vi "TestFileCreationAndWriting.vi"() -> ()   [LabVIEW 2014]
panel:
  in  "VME Configuration":T1={"Module Description"=["Bridge", "TDC", "Scaler", "Hodoscope QDC ", "Other QDC", "Digitizer 1", "Digitizer 2", ""], "Module Model"=["V2718", "V775", "V830", "V965A", "V965A", "V1729A", "1729A", ""], "Module Address"=[0, 4026597376, 4026662912, 4026728448, 4026793984, 4026859520, 4026925056]} {"Module Address" format="%.0x"}
  out "error out":errorcluster
  out "Average Write Time (ms)":dbl=11.54
  out "Max Write Time":u32=42
  in  "Number of Events":i32=100
  in  "QDC Info":T2={"Chanel Description"=["H0", "H1", "H2", "H3", "H4", "H5"], "Only Hodo?"=[TRUE, TRUE, TRUE, TRUE, TRUE, TRUE]}
  in  "Scaler Info":T2={"Chanel Description"=["H0", "H1", "H2", "H3", "H4", "H5", "TrigA", "TrigB", "TrigC", "TrigD", "Ch0", "Ch1", "Ch2", "Ch3", "Ch4", "Ch5", "Ch6", "Ch7"], "Only Hodo?"=[TRUE, TRUE, TRUE, TRUE, TRUE, TRUE, TRUE, TRUE, FALSE, FALSE, FALSE, FALSE, FALSE, FALSE, FALSE, FALSE, FALSE, FALSE]}
  in  "Digitizer Info":T2={"Chanel Description"=["Ch0", "Ch1", "Ch2", "Ch3", "Ch4", "Ch5", "Ch6", "Ch7"], "Only Hodo?"=[FALSE, FALSE, FALSE, FALSE, FALSE, FALSE, FALSE, FALSE]}
  in  "TDC Info":T2={"Chanel Description"=["H0", "H1", "H2", "H3", "H4", "H5", "TrigA", "TrigB", "TrigC", "TrigD"], "Only Hodo?"=[TRUE, TRUE, TRUE, TRUE, TRUE, TRUE, TRUE, TRUE, FALSE, FALSE]}
  in  "Trigger Bit Descriptions":string[](array[string])=["TrigA", "TrigB", "TrigC", "TrigD"]
  in  "Thermocouple Location":string[](array[string])=["In Dark Box", "In Room"]
  in  "HDF5 File Path":path=path "C:/Users/lbignell/Desktop/Control Software/HDF5/Dummy3.h5"
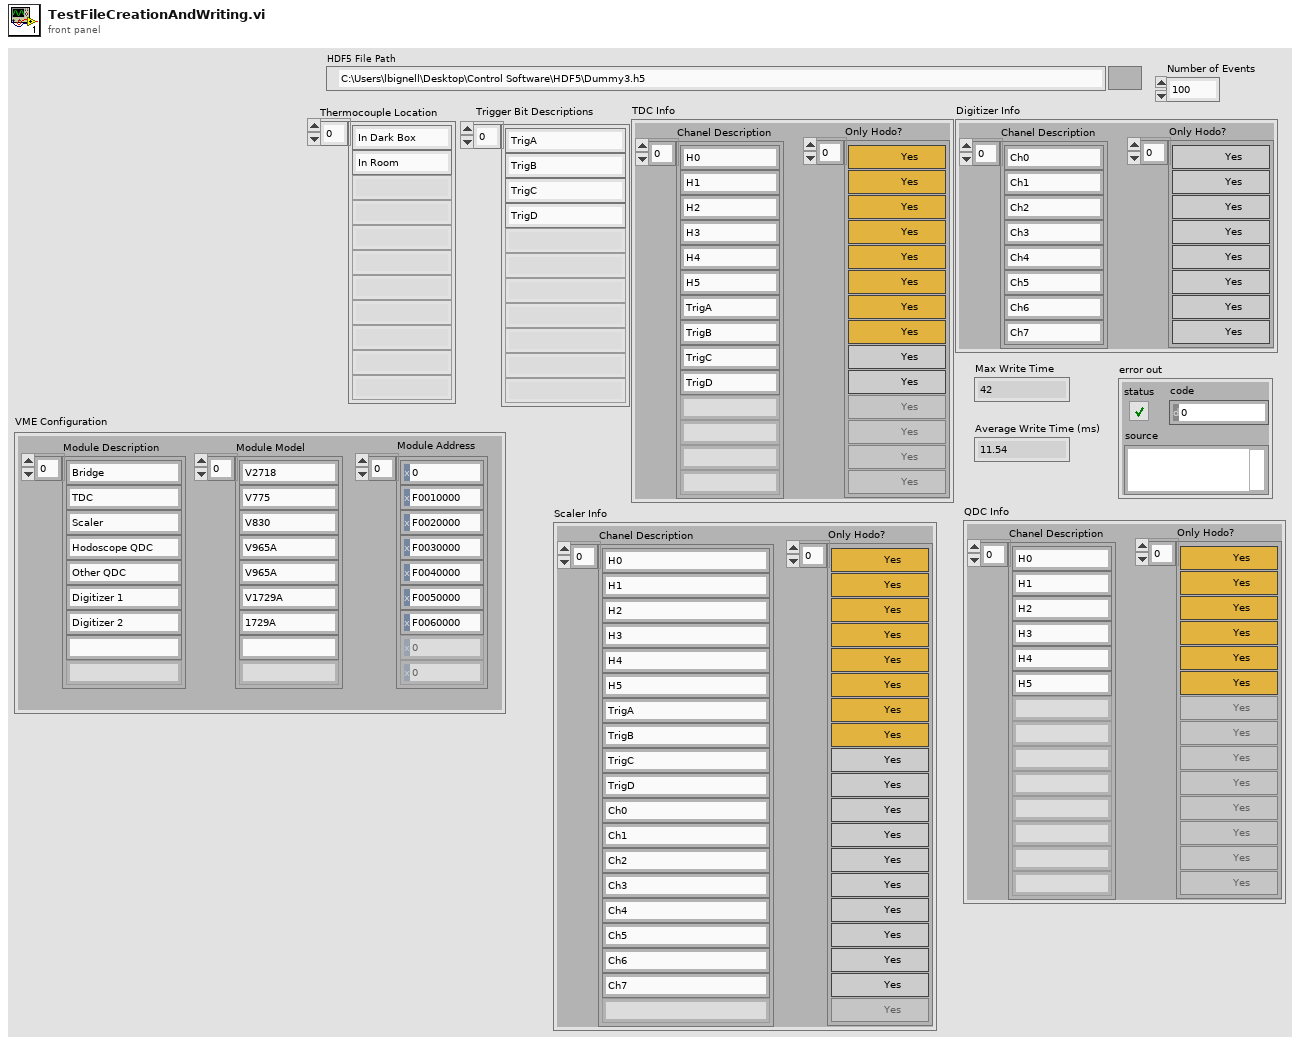
[diagram p1: front panel]
types:
  T1 = cluster{"Module Description":string[], "Module Model":string[], "Module Address":u32[]}
  T2 = cluster{"Chanel Description":string[], "Only Hodo?":bool[]}
  T3 = typedef "hid_t.ctl" = i32
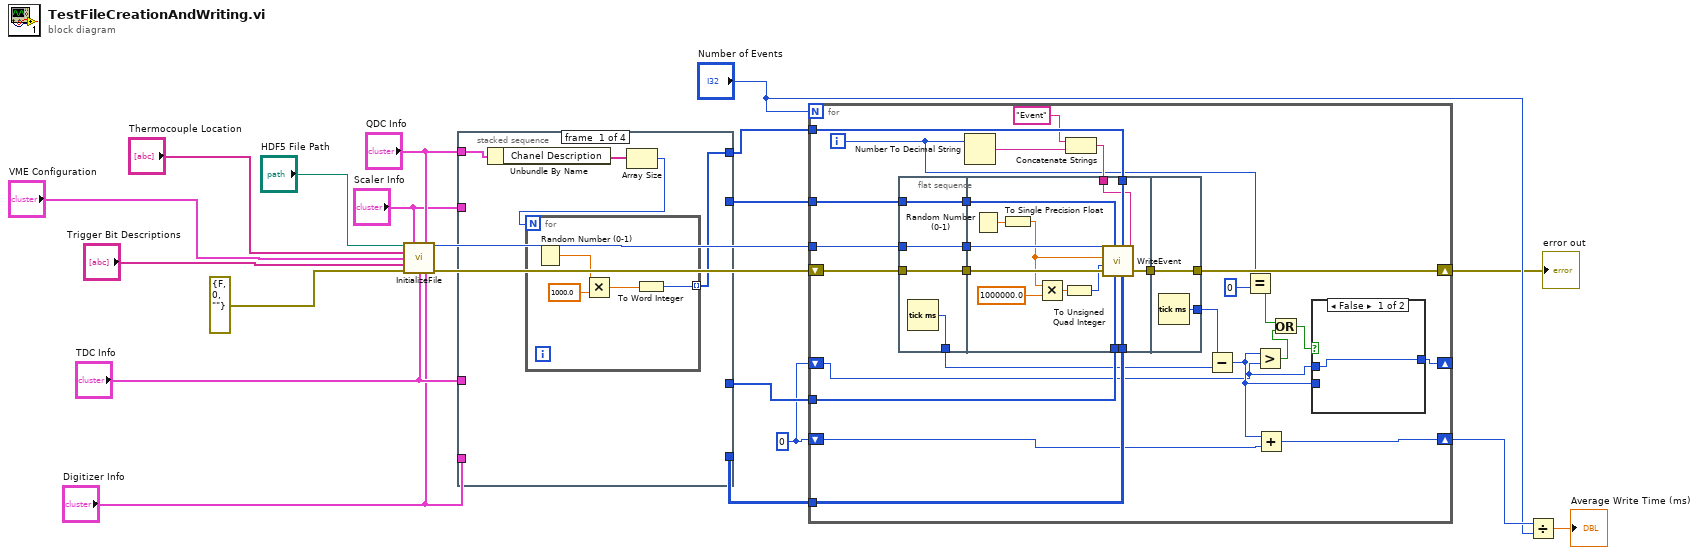
[diagram p0: block diagram]
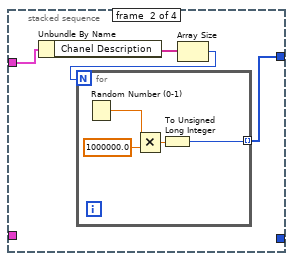
[diagram p2: hidden frame]
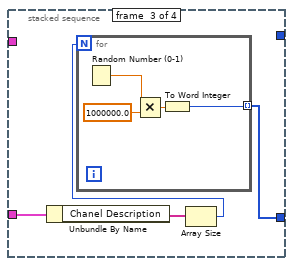
[diagram p3: hidden frame]
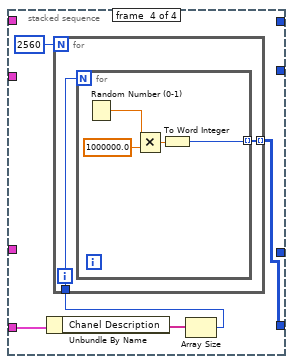
[diagram p4: hidden frame]
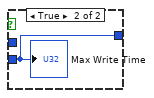
[diagram p5: hidden frame]
diagram:
  w2 = u32 0
  n1 = call "InitializeFile.vi"("File Path"="HDF5 File Path", "Scaler Info"="Scaler Info", "QDC Info"="QDC Info", "Thermocouple Location"="Thermocouple Location", "VME Configuration"="VME Configuration", "Trigger Bit Descriptions"="Trigger Bit Descriptions", "error in"=errorcluster {"status"=FALSE, "code"=0, "source"=""}, "TDC Info"="TDC Info", "Digitizer Info"="Digitizer Info") -> ("File Handle"=w16:T3, "error out"=w7:errorcluster)  [unwired: 5 in]
  n2 = stacked-sequence {
    tunnel: "QDC Info" -> [w24 _ _ _]
    tunnel: [w21 _ _ _] -> w14
    tunnel: "Scaler Info" -> [_ w30 _ _]
    tunnel: [_ w29 _ _] -> w12
    tunnel: "TDC Info" -> [_ _ w38 _]
    tunnel: [_ _ w37 _] -> w10
    tunnel: "Digitizer Info" -> [_ _ _ w47]
    tunnel: [_ _ _ w45] -> w8
    frame #0 {
      n3 = Unbundle By Name(w24) -> ("Chanel Description"=w23:string[])
      n4 = Array Size(array=w23) -> (size(s)=w22:i32)
      n5 = for {
        N: w22 -> [_]
        tunnel: [w25] -> w21 mode=indexing
        n6 = Random Number (0-1)() -> (number: 0 to 1=w27:dbl)
        n7 = Multiply(x=w27, y=1000.0) -> (x*y=w26:dbl)
        n8 = To Word Integer(number=w26) -> (16bit integer=w25:i16)
      }
    }
    frame #1 {
      n9 = Unbundle By Name(w30) -> ("Chanel Description"=w32:string[])
      n10 = Array Size(array=w32) -> (size(s)=w31:i32)
      n11 = for {
        N: w31 -> [_]
        tunnel: [w33] -> w29 mode=indexing
        n12 = Random Number (0-1)() -> (number: 0 to 1=w35:dbl)
        n13 = Multiply(x=w35, y=1000000.0) -> (x*y=w34:dbl)
        n14 = To Unsigned Long Integer(number=w34) -> (unsigned 32bit integer=w33:u32)
      }
    }
    frame #2 {
      n15 = Unbundle By Name(w38) -> ("Chanel Description"=w40:string[])
      n16 = Array Size(array=w40) -> (size(s)=w39:i32)
      n17 = for {
        N: w39 -> [_]
        tunnel: [w41] -> w37 mode=indexing
        n18 = Random Number (0-1)() -> (number: 0 to 1=w43:dbl)
        n19 = Multiply(x=w43, y=1000000.0) -> (x*y=w42:dbl)
        n20 = To Word Integer(number=w42) -> (16bit integer=w41:i16)
      }
    }
    frame #3 {
      n21 = Unbundle By Name(w47) -> ("Chanel Description"=w49:string[])
      n22 = Array Size(array=w49) -> (size(s)=w48:i32)
      n23 = for {
        N: 2560 -> [_]
        tunnel: w48 -> [w51]
        tunnel: [w50] -> w45 mode=indexing
        n24 = for {
          N: w51 -> [_]
          tunnel: [w52] -> w50 mode=indexing
          n25 = Random Number (0-1)() -> (number: 0 to 1=w54:dbl)
          n26 = Multiply(x=w54, y=1000000.0) -> (x*y=w53:dbl)
          n27 = To Word Integer(number=w53) -> (16bit integer=w52:i16)
        }
      }
    }
  }
  n28 = for {
    N: "Number of Events" -> [_]
    tunnel: w16 -> [w81]
    tunnel: w14 -> [w80]
    tunnel: w12 -> [w79]
    tunnel: w10 -> [w78]
    tunnel: w8 -> [w77]
    shift-right: [w71] -> w6
    shift-left: w2 -> [w69]
    shift-right: [w72] -> w3
    shift-left: w7 -> [w70]
    shift-right: [w61] -> _
    shift-left: w2 -> [w56]
    i -> [w62]
    n29 = flat-sequence {
      tunnel: w79 -> [w85]
      tunnel: w81 -> [w86]
      tunnel: w70 -> [w87]
      tunnel: [w87] -> w76
      tunnel: [w86] -> w75
      tunnel: [w85] -> w74
      tunnel: [w84] -> w64
      tunnel: w80 -> [w93]
      tunnel: w78 -> [w91]
      tunnel: w77 -> [w90]
      tunnel: w76 -> [w100]
      tunnel: w75 -> [w99]
      tunnel: w74 -> [w92]
      tunnel: [w89] -> w73
      tunnel: w66 -> [w88]
      tunnel: w73 -> [w102]
      tunnel: [w102] -> w72
      tunnel: [w101] -> w65
      frame #0 {
        n30 = Tick Count (ms)() -> (millisecond timer value=w84:u32)
      }
      frame #1 {
        n31 = Random Number (0-1)() -> (number: 0 to 1=w98:dbl)
        n32 = To Single Precision Float(number=w98) -> (single precision float=w94:sgl)
        n33 = Multiply(x=w94, y=1000000.0) -> (x*y=w96:dbl)
        n34 = To Unsigned Quad Integer(1:w96) -> (0:w95:u64)
        n35 = call "WriteEvent.vi"("Evt name"=w88, "Digitizer Data"=w90, "QDC Data"=w93, "TDC Data"=w91, "Scaler Data"=w92, "error in"=w100, "Trigger Bits (as U64)"=w95, "Temperature"=w94, "file ref in"=w99) -> ("error out"=w89:errorcluster)  [unwired: 2 in]
      }
      frame #2 {
        n36 = Tick Count (ms)() -> (millisecond timer value=w101:u32)
      }
    }
    n37 = Number To Decimal String(number=w62) -> (decimal integer string=w67:string)  [unwired: 1 in]
    n38 = Concatenate Strings("Event", w67) -> (w66:string)
    n39 = Subtract(x=w65, y=w64) -> (x-y=w60:u32)
    n40 = Equal?(x=w62, y=0) -> (x = y?=w58:bool)
    n41 = Greater?(x=w60, y=w56) -> (0:w59:bool)
    n42 = Add(x=w60, y=w69) -> (x+y=w71:u32)
    n43 = Or(x=w58, y=w59) -> (x .or. y?=w57:bool)
    n44 = case shown="False" w57 {
      tunnel: w60 -> [_ w83]
      tunnel: [w82 w83] -> w61
      tunnel: w56 -> [w82 _]
      frame False {
      }
      frame True {
        "Max Write Time" <- w83
      }
    }
  }
  "error out" <- w3
  n45 = Divide(x=w6, y="Number of Events") -> (x/y=→"Average Write Time (ms)":dbl)
